vi "Diameter to Area.vi"(11 "Diameter (m)":dbl) -> (3 "Area (m^2)":dbl)   [LabVIEW 2019]
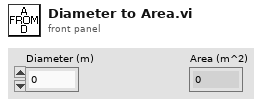
[diagram p1: front panel]
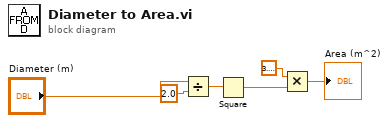
[diagram p0: block diagram]
diagram:
  n1 = Divide(x="Diameter (m)", y=2.0) -> (x/y=w3:dbl)
  n2 = Square(x=w3) -> (x^2=w4:dbl)
  n3 = Multiply(x=3.141592653589793, y=w4) -> (x*y=→"Area (m^2)":dbl)
